vi "Create.vi"(10 "Task ID":string) -> (3 "DataLoggerIdentity out":refnum<class "DataLoggerIdentity.lvclass">)   [LabVIEW 2020, in "VolatusData.lvlib" / "DataLoggerIdentity.lvclass"]
uses:
  DataLoggerIdentity.lvclass
  DataLoggerIdentity.lvclass/DataLoggerIdentity.ctl
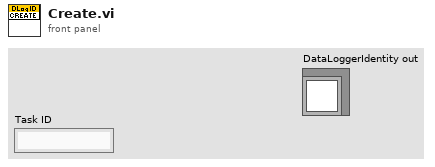
[diagram p1: front panel]
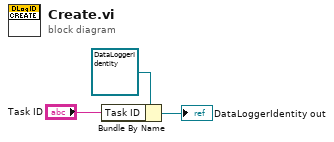
[diagram p0: block diagram]
diagram:
  n1 = Bundle By Name(cluster=refnum<class "DataLoggerIdentity.lvclass"> refnum ("DataLoggerIdentity in"), "Task ID"="Task ID") -> (→"DataLoggerIdentity out":refnum<class "DataLoggerIdentity.lvclass">)
